vi "_VISA_Allocator.vi"(8 "error in (no error)":errorcluster, 9 "Master done":bool, 10 "Master requester":bool) -> (0 "error out":errorcluster, 1 "Master done?":bool, 3 "VISA out":refnum<visa-resource-name>)   [LabVIEW 2016]
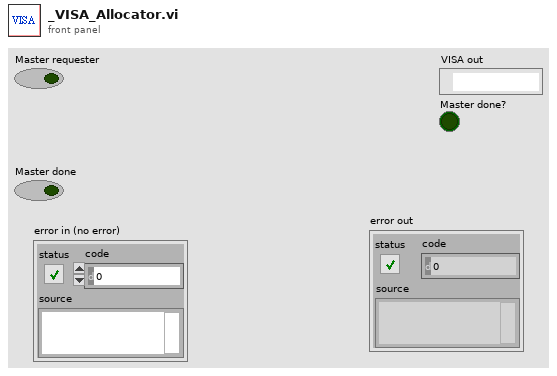
[diagram p1: front panel]
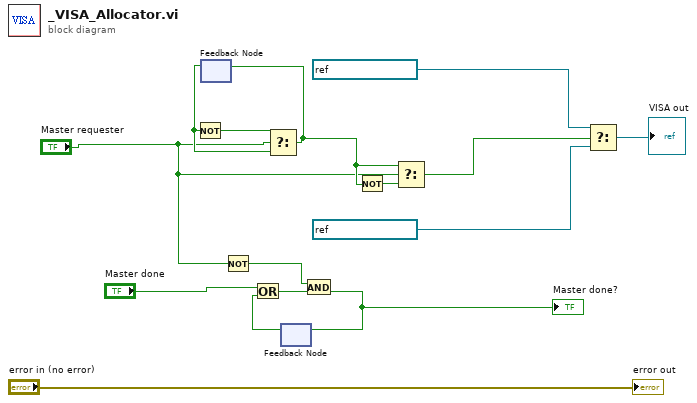
[diagram p0: block diagram]
diagram:
  n1 = feedback #1() -> (w14:bool)  [unwired: 1 in]
  n2 = Not(x=w14) -> (.not. x?=w15:bool)
  n3 = Not(x="Master requester") -> (.not. x?=w1:bool)
  n4 = Select(t=w15, s="Master requester", f=w14) -> (s? t:f=w9:bool)
  n5 = feedback-in #1(w9) -> ()
  n6 = feedback #2() -> (w4:bool)  [unwired: 1 in]
  n7 = Or(x="Master done", y=w4) -> (x .or. y?=w5:bool)
  n8 = And(x=w1, y=w5) -> (x .and. y?=w3:bool)
  "Master done?" <- w3
  n9 = feedback-in #2(w3) -> ()
  n10 = Not(x=w9) -> (.not. x?=w8:bool)
  n11 = Select(t=w9, s="Master requester", f=w8) -> (s? t:f=w10:bool)
  n12 = Select(t=refnum<visa-resource-name> "ASRL1::INSTR" ("VISA resource name"), s=w10, f=refnum<visa-resource-name> "ASRL2::INSTR" ("VISA resource name")) -> (s? t:f=→"VISA out":refnum<visa-resource-name>)
  "error out" <- "error in (no error)"
